vi "Get SRS785 status.vi"(8 "error in (no error)":errorcluster, 11 "VISA resource name":refnum<visa-resource-name>) -> (0 "error out":errorcluster, 2 "concatenated string":string, 3 "VISA resource name out":refnum<visa-resource-name>, 4 "Fre multipler kHz":ext, 5 "Center frequency":dbl, 6 "Fre start kHz":dbl, 7 "Frequency Span":dbl)   [LabVIEW 2023]
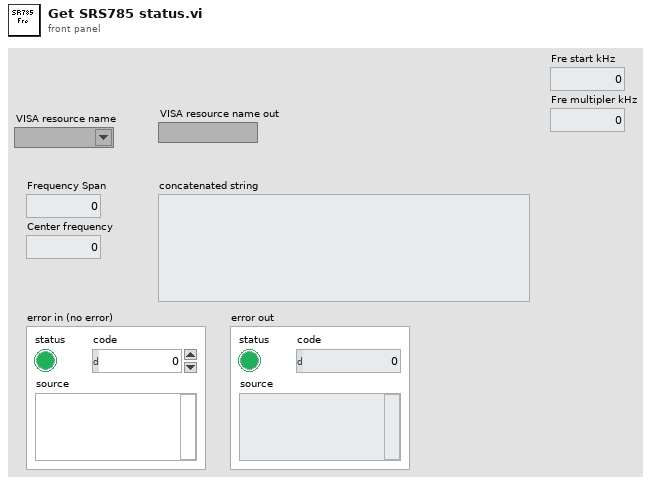
[diagram p1: front panel]
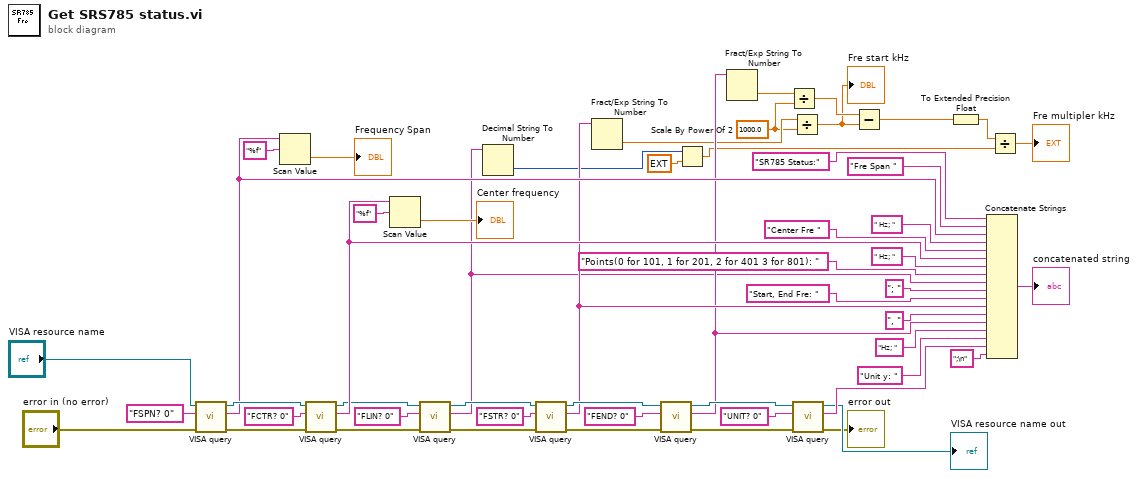
[diagram p0: block diagram]
diagram:
  w10 = 1000.0 ("y")
  n1 = call "VISA query.vi"("error in (no error)"="error in (no error)", "write buffer"="FSPN? 0", "VISA Refnum in"="VISA resource name") -> ("error out"=w49:errorcluster, "read buffer"=w15:string, "VISA Refnum out"=w48:refnum<visa-resource-name>)  [unwired: 6 in]
  n2 = Scan Value(string=w15, format string="%f") -> (value=→"Frequency Span":dbl)  [unwired: 1 in, 1 out]
  n3 = call "VISA query.vi"("error in (no error)"=w49, "write buffer"="FCTR? 0", "VISA Refnum in"=w48) -> ("error out"=w36:errorcluster, "read buffer"=w40:string, "VISA Refnum out"=w37:refnum<visa-resource-name>)  [unwired: 6 in]
  n4 = Scan Value(string=w40, format string="%f") -> (value=→"Center frequency":dbl)  [unwired: 1 in, 1 out]
  n5 = call "VISA query.vi"("error in (no error)"=w36, "write buffer"="FLIN? 0", "VISA Refnum in"=w37) -> ("error out"=w31:errorcluster, "read buffer"=w6:string, "VISA Refnum out"=w32:refnum<visa-resource-name>)  [unwired: 6 in]
  n6 = Decimal String To Number(string=w6) -> (number=w5:i32)  [unwired: 2 in, 1 out]
  n7 = call "VISA query.vi"("error in (no error)"=w31, "write buffer"="FSTR? 0", "VISA Refnum in"=w32) -> ("error out"=w28:errorcluster, "read buffer"=w14:string, "VISA Refnum out"=w29:refnum<visa-resource-name>)  [unwired: 6 in]
  n8 = Fract/Exp String To Number(string=w14) -> (number=w12:dbl)  [unwired: 3 in, 1 out]
  n9 = call "VISA query.vi"("error in (no error)"=w28, "write buffer"="FEND? 0", "VISA Refnum in"=w29) -> ("error out"=w22:errorcluster, "read buffer"=w13:string, "VISA Refnum out"=w23:refnum<visa-resource-name>)  [unwired: 6 in]
  n10 = Scale By Power Of 2(n=w5, x=ext 100.0) -> (x*2^n=w3:ext)
  n11 = Fract/Exp String To Number(string=w13) -> (number=w11:dbl)  [unwired: 3 in, 1 out]
  n12 = Divide(x=w11, y=w10) -> (x/y=w9:dbl)
  n13 = Divide(x=w12, y=w10) -> (x/y=w8:dbl)
  "Fre start kHz" <- w8
  n14 = call "VISA query.vi"("error in (no error)"=w22, "write buffer"="UNIT? 0", "VISA Refnum in"=w23) -> ("error out"=→"error out":errorcluster, "read buffer"=w19:string, "VISA Refnum out"=→"VISA resource name out":refnum<visa-resource-name>)  [unwired: 6 in]
  n15 = Subtract(x=w9, y=w8) -> (x-y=w7:dbl)
  n16 = To Extended Precision Float(1:w7) -> (0:w2:ext)
  n17 = Concatenate Strings("SR785 Status:" ("string"), "Fre Span " ("string"), w15, " Hz; " ("string"), "Center Fre " ("string"), w40, " Hz; " ("string"), "Points(0 for 101, 1 for 201, 2 for 401 3 for 801): " ("string"), w6, "; " ("string"), "Start, End Fre: " ("string"), w14, ", " ("string"), w13, "Hz; " ("string"), "Unit y: " ("string"), w19, ";\n" ("string")) -> (→"concatenated string":string)
  n18 = Divide(x=w2, y=w3) -> (x/y=→"Fre multipler kHz":ext)
